vi "Close VI.vi"(10 "VI Refnum":refnum<vi>, 11 "App Ref":refnum<vi>) -> ()   [LabVIEW 2024, in "Wordle Scorer.lvlib"]
uses:
  Wordle Scorer.lvlib
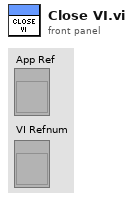
[diagram p1: front panel]
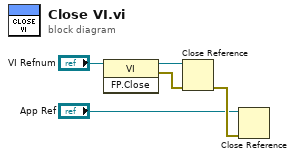
[diagram p0: block diagram]
diagram:
  n1 = invoke class="VI" method="FP.Close"(reference="VI Refnum") -> (reference out=w3:refnum<vi>, error out=w2:errorcluster)  [unwired: 2 in, 1 out]
  n2 = Close Reference(reference=w3, error in (no error)=w2) -> (error out=w5:errorcluster)
  n3 = Close Reference(reference="App Ref", error in (no error)=w5) -> ()  [unwired: 1 out]
